vi "Zustands Logger.vi"   [LabVIEW 2020, in "Funktionstasten.lvlib"]
uses:
  Funktionstasten.lvlib
  Seiten/System Einstellungen V2/Aktioen FGV System.ctl
  Aktionen Zustaende Loggen.ctl
  Allgemein/allgemeine Sub-VIs.lvlib
  Seiten/System Einstellungen V2/System Einstellungen V2.lvlib
panel:
  # "Zustandswechsel in Datei loggen!"
types:
  T1 = typedef "System Einstellungen V2.lvlib/Aktioen FGV System.ctl" = enum16{"lesen", "laden", "speichern", "Optionen schreiben", "Zeitstempel", "Reset BMP", "Reset SQP", "Wartung", "Werkseinstellung"}
  T2 = typedef "System Einstellungen V2.lvlib/Optionen.ctl" = cluster{"Störmeldep.":bool, "Betriebszustände":bool, "AK in ppm":bool, "log Cal-Gas":bool, "log 0-Gas":bool, "Durchflusssensor 0-5V":bool, "PNS?":bool, "Mit N2 spülen":bool, "TRE08":bool, "Amium 10-Fach":bool, "Verticale Scrollbar aktiv":bool, "Loggingtakt":bool, "AK Rezeptwechsel gleich wie MKS":bool, "NG ECO":bool}
  T3 = typedef "Funktionstasten.lvlib/Aktionen Zustaende Loggen.ctl" = enum16{"lesen", "schreiben", "löschen", "init"}
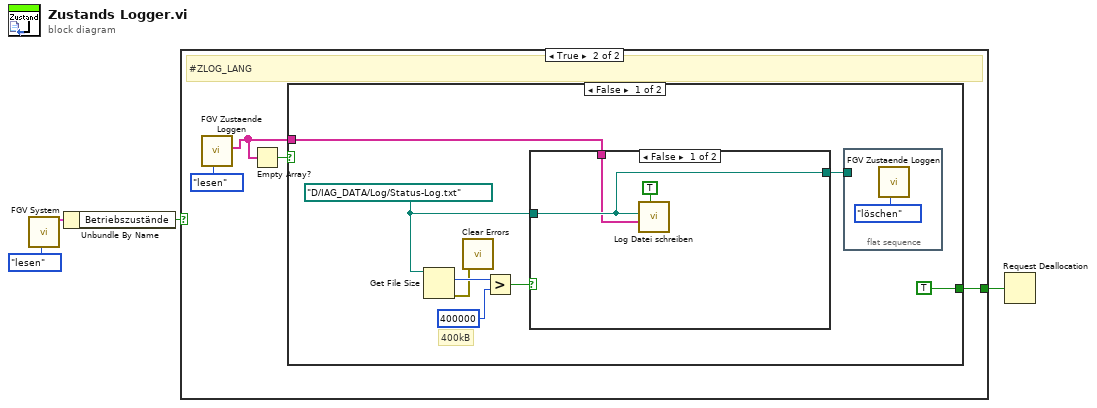
[diagram p0: block diagram]
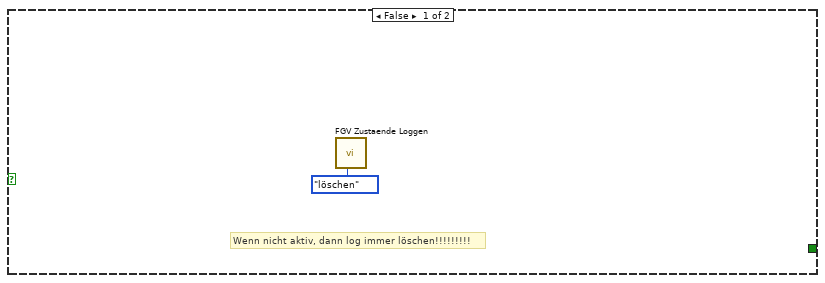
[diagram p2: hidden frame]
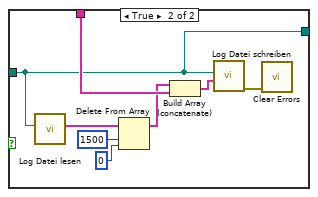
[diagram p3: hidden frame]
diagram:
  n1 = call "FGV System.vi"("Aktionen"=Aktioen_FGV_System."lesen") -> ("Optionen"=w3:T2)  [unwired: 12 in, 6 out]
  n2 = Unbundle By Name(w3) -> ("Betriebszustände"=w2:bool)
  n3 = case shown="True" w2 {
    tunnel: [_ w7] -> w1
    frame False {
      # "Wenn nicht aktiv, dann log immer löschen!!!!!!!!!"
      n4 = call "FGV Zustaende Loggen.vi"("Aktionen Zustände Loggen"=Aktionen_Zustaende_Loggen."löschen") -> ()  [unwired: 9 in, 2 out]
    }
    frame True {
      # "#ZLOG_LANG"
      n5 = call "FGV Zustaende Loggen.vi"("Aktionen Zustände Loggen"=Aktionen_Zustaende_Loggen."lesen") -> ("Log Daten Lang"=w6:string[])  [unwired: 9 in, 1 out]
      n6 = Empty Array?(array=w6) -> (empty?=w9:bool)
      n7 = case shown="False" w9 {
        tunnel: w6 -> [w12 _]
        tunnel: [TRUE _] -> w7
        frame False {
          w14 = path "D:/IAG_DATA/Log/Status-Log.txt" ("Datei")
          # "400kB"
          n8 = Get File Size(file=w14) -> (size (in bytes)=w15:i64, 0:w13:errorcluster)  [unwired: 1 in, 1 out]
          n9 = call <vilib>:"Clear Errors.vi"("error in (no error)"=w13) -> ()  [unwired: 5 in, 2 out]
          n10 = Greater?(x=w15, y=i64 400000) -> (0:w17:bool)
          n11 = case shown="False" w17 {
            tunnel: w12 -> [w20 w28]
            tunnel: w14 -> [w21 w25]
            tunnel: [w21 w25] -> w11
            frame False {
              n12 = call "Log Datei schreiben.vi"("An Datei Anhängen?"=TRUE, "Array"=w20, "Dateipfad"=w21) -> ()  [unwired: 8 in, 1 out]
            }
            frame True {
              n13 = call "Log Datei lesen.vi"("Dateipfad"=w25) -> ("Array"=w26:string[])  [unwired: 10 in]
              n14 = Delete From Array(array=w26, length=1500 ("Länge"), index=0 ("Index")) -> (array with subset deleted=w27:string[])  [unwired: 1 out]
              n15 = Build Array (concatenate)(w27, w28) -> (w24:string[])
              n16 = call "Log Datei schreiben.vi"("Array"=w24, "Dateipfad"=w25) -> ("error out"=w23:errorcluster)  [unwired: 9 in]
              n17 = call <vilib>:"Clear Errors.vi"("error in (no error)"=w23) -> ()  [unwired: 5 in, 2 out]
            }
          }
          n18 = flat-sequence {
            tunnel: [w18] -> _
            tunnel: w11 -> [w18]
            frame #0 {
              n19 = call "FGV Zustaende Loggen.vi"("Aktionen Zustände Loggen"=Aktionen_Zustaende_Loggen."löschen") -> ()  [unwired: 9 in, 2 out]
            }
          }
        }
        frame True {
        }
      }
    }
  }
  n20 = Request Deallocation(w1) -> ()
